vi "Get Missing Required Options.vi"(8 "error in (no error)":errorcluster, 11 "Options":refnum<class "Option.lvclass">[](array[class])) -> (0 "error out":errorcluster, 2 "Missing Keys":string[](array[string]))   [LabVIEW 2011, in "Option Parser.lvlib" / "Option Set.lvclass"]
doc: "Get Missing Required Options"
uses:
  Option Set.lvclass
  Option Class/Option.lvclass
  Option Class/Read Key.vi
  Option Class/Read Required.vi
  Option Class/Read Set.vi
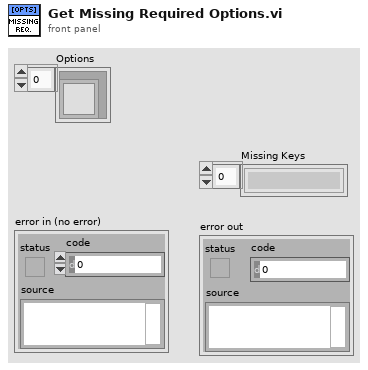
[diagram p1: front panel]
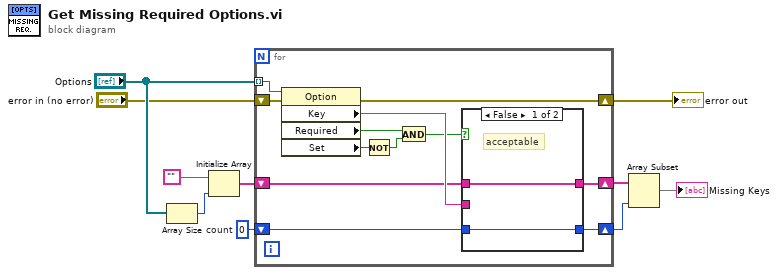
[diagram p0: block diagram]
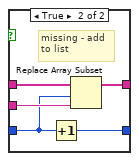
[diagram p2: hidden frame]
diagram:
  w10 = 0  # count
  n1 = Array Size(array="Options") -> (size(s)=w9:i32)
  n2 = Initialize Array("", w9) -> (w7:string[])
  n3 = for {
    tunnel: "Options" -> [w20] mode=indexing
    shift-right: [w21] -> w5
    shift-left: "error in (no error)" -> [w22]
    shift-right: [w16] -> w3
    shift-left: w7 -> [w14]
    shift-right: [w12] -> w1
    shift-left: w10 -> [w13]
    n4 = property class="Option"(reference=w20, error in=w22) -> (error out=w21:errorcluster, "Key"=w15:string, "Required"=w17:bool, "Set"=w19:bool)  [unwired: 1 out]
    n5 = Not(x=w19) -> (.not. x?=w18:bool)
    n6 = And(x=w17, y=w18) -> (x .and. y?=w11:bool)
    n7 = case shown="False" w11 {
      tunnel: [w24 w29] -> w16
      tunnel: w15 -> [_ w28]
      tunnel: w14 -> [w24 w27]
      tunnel: w13 -> [w23 w26]
      tunnel: [w23 w25] -> w12
      frame False {
        # "acceptable"
      }
      frame True {
        # "missing - add\nto list"
        n8 = Increment(x=w26) -> (x+1=w25:i32)
        n9 = Replace Array Subset(array=w27, new element=w28, index=w26) -> (w29:string[])
      }
    }
  }
  "error out" <- w5
  n10 = Array Subset(array=w3, length=w1) -> (→"Missing Keys":string[])  [unwired: 1 in]
